vi "Create.vi"(10 "Groups":refnum<class "Group.lvclass">[](array[class])) -> (3 "GroupsAbstractValue out":refnum<class "GroupsAbstractValue.lvclass">)   [LabVIEW 2020, in "Vecto.lvlib" / "GroupsAbstractValue.lvclass"]
uses:
  GroupsAbstractValue.lvclass
  Group/Group.lvclass
  GroupsAbstractValue.lvclass/GroupsAbstractValue.ctl
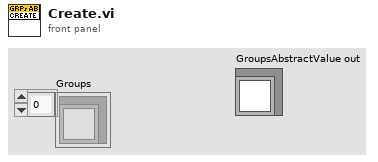
[diagram p1: front panel]
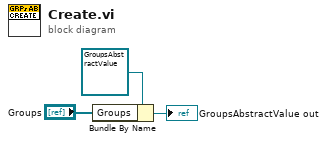
[diagram p0: block diagram]
diagram:
  n1 = Bundle By Name(cluster=refnum<class "GroupsAbstractValue.lvclass"> refnum ("GroupsAbstractValue in"), "Groups"="Groups") -> (→"GroupsAbstractValue out":refnum<class "GroupsAbstractValue.lvclass">)
